vi "CD Init_Prepare Async Data_RT Command Channels.vi"(8 "error in (no error)":errorcluster, 10 "Card Parameters (in)":T1, 11 "Channels In":T6[](array[typedef]) {"RTs"."Mode Codes"."Words Item Refs" format="%.0x"; "RTs"."Mode Codes"."Timestamp Channel Data Reference" format="%.0x"; "RTs"."subAddresses"."Words Item Refs" format="%.0x"; "RTs"."subAddresses"."Timestamp Channel Data Reference" format="%.0x"; "RTs"."Status Channel Data Reference" format="%.0x"; "RTs"."Command Channels Refs" format="%.0x"; "BC"."Acyclic Frames Trigger Channels Refs" format="%.0x"; "BC"."Command Channels Refs" format="%.0x"; "BC"."messages"."Timestamp Channel Data Reference" format="%.0x"; "BC"."messages"."Status Channel Data Refs" format="%.0x"; "BC"."messages"."Words Item Refs" format="%.0x"; "BC"."messages"."Words Block Data Refs"."Data Reference" format="%.0x"}) -> (0 "error out":errorcluster, 3 "Map (RT Command Channels)":T3[](array[typedef]) {"RT Command Channel Ref" format="%.0x"})   [LabVIEW 2017, in "Ballard MIL-1553 Engine.lvlib"]
doc: "This VI creates a static association between NI-VS FIFO Channel Index and Physical Channel, Label Index, Parameter Index for Parameter Channel of a Tx Scheduled Label."
uses:
  Ballard MIL-1553 Engine.lvlib
  Shared/Controls and Global/RT Channel.ctl
  Shared/Controls and Global/RT BC.ctl
  <vilib>/NI Veristand/Custom Device API/Custom Device Item Ref.ctl
  Shared/Controls and Global/RT Message.ctl
  Shared/Controls and Global/RT messageType.ctl
  Shared/Controls and Global/RT CWD1.ctl
  Shared/Controls and Global/RT CWD2.ctl
  <vilib>/NI Veristand/Custom Device API/Data Reference.ctl
  <vilib>/NI Veristand/Custom Device API/Block Data Reference.ctl
  Shared/Controls and Global/RT Remote Terminal.ctl
  Shared/Controls and Global/RT Remote Terminal_rtMode.ctl
  Shared/Controls and Global/RT Remote Terminal_RT subAddress.ctl
  Shared/Controls and Global/RT Remote Terminal_RT direction.ctl
  Shared/Controls and Global/RT Remote Terminal_RT Mode Code.ctl
  Controls/RT Async_Map RT Command Channels.ctl
  Controls/RT Async_Map_Type.ctl
  Controls/Card Parameters.ctl
  Shared/Controls and Global/Initialization Method.ctl
  <vilib>/NI VeriStand/Custom Device API/Custom Device API.lvlib
  <instrlib>/BTI1553Lib/BTI1553LV.lvlib
  Shared/Ballard 1553 Shared.lvlib
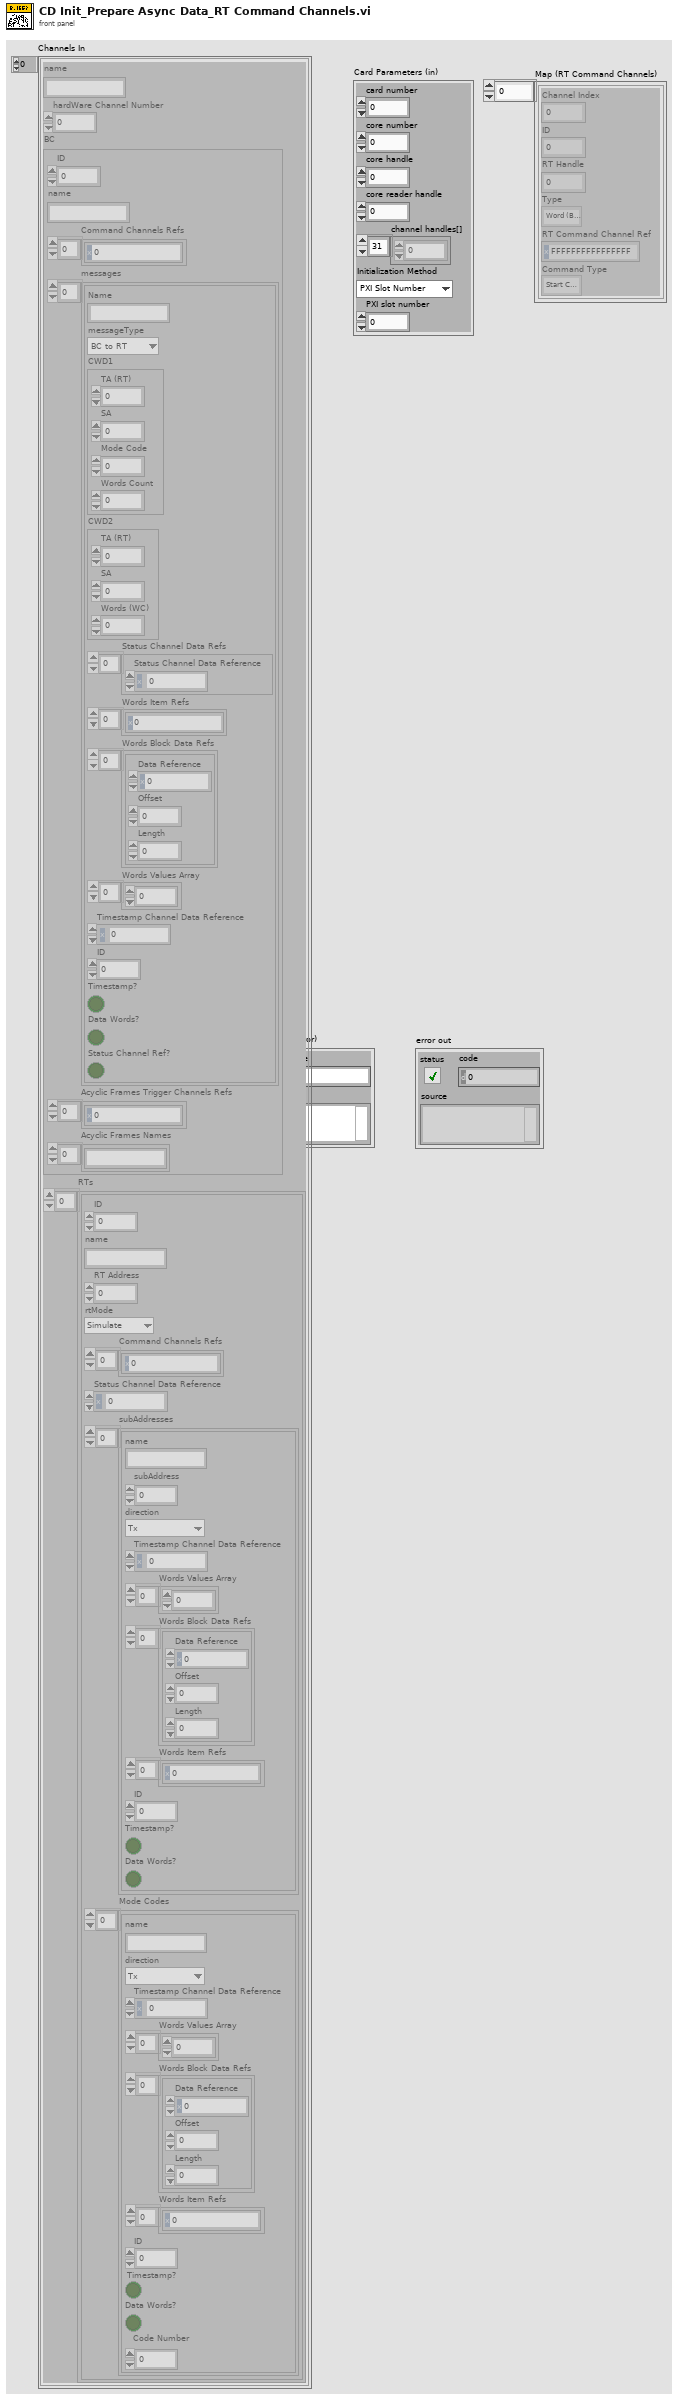
[diagram p1: front panel]
types:
  T1 = typedef "Ballard MIL-1553 Engine.lvlib/Card Parameters.ctl" = cluster{"card number":i32, "core number":i32, "core handle":u64, "core reader handle":u64, "channel handles[]":u64[], "Initialization Method":T2, "PXI slot number":i32}
  T2 = typedef "Ballard 1553 Shared.lvlib/Initialization Method.ctl" = enum16{"PXI Slot Number", "Card Number"}
  T3 = typedef "Ballard MIL-1553 Engine.lvlib/RT Async_Map RT Command Channels.ctl" = cluster{"Channel Index":i32, "ID":i32, "RT Handle":u64, "Type":T4, "RT Command Channel Ref":T5, "Command Type":enum16{"Start Command", "Stop Command"}}
  T4 = typedef "Ballard MIL-1553 Engine.lvlib/RT Async_Map_Type.ctl" = enum16{"Word (BC to RT)", "Word (MC (Rx))", "Acyclic Message Trigger", "Word (RT to ..)", "Word (RT to RT)", "Word (MC (Tx))", "RT Status", "BC Commands", "RT Commands"}
  T5 = typedef "Custom Device API.lvlib/Custom Device Item Ref.ctl" = u64
  T6 = typedef "Ballard 1553 Shared.lvlib/RT Channel.ctl" = cluster{"name":string, "hardWare Channel Number":u16, "BC":T7, "RTs":T14[]}
  T7 = typedef "Ballard 1553 Shared.lvlib/RT BC.ctl" = cluster{"ID":i32, "name":string, "Command Channels Refs":T5[], "messages":T8[], "Acyclic Frames Trigger Channels Refs":T5[], "Acyclic Frames Names":string[]}
  T8 = typedef "Ballard 1553 Shared.lvlib/RT Message.ctl" = cluster{"Name":string, "messageType":T9, "CWD1":T10, "CWD2":T11, "Status Channel Data Refs":T12[], "Words Item Refs":T5[], "Words Block Data Refs":T13[], "Words Values Array":u16[], "Timestamp Channel Data Reference":T12, "ID":i32, "Timestamp?":bool, "Data Words?":bool, "Status Channel Ref?":bool}
  T9 = typedef "Ballard 1553 Shared.lvlib/RT messageType.ctl" = enum16{"BC to RT", "RT to BC", "RT to RT", "MC (Rx)", "MC (Tx)"}
  T10 = typedef "Ballard 1553 Shared.lvlib/RT CWD1.ctl" = cluster{"TA (RT)":i8, "SA":i8, "Mode Code":i8, "Words Count":i8}
  T11 = typedef "Ballard 1553 Shared.lvlib/RT CWD2.ctl" = cluster{"TA (RT)":i8, "SA":i8, "Words (WC)":i8}
  T12 = typedef "Custom Device API.lvlib/Data Reference.ctl" = i32
  T13 = typedef "Custom Device API.lvlib/Block Data Reference.ctl" = cluster{"Data Reference":T12, "Offset":u64, "Length":u64}
  T14 = typedef "Ballard 1553 Shared.lvlib/RT Remote Terminal.ctl" = cluster{"ID":i32, "name":string, "RT Address":i32, "rtMode":T15, "Command Channels Refs":T5[], "Status Channel Data Reference":T12, "subAddresses":T16[], "Mode Codes":T18[]}
  T15 = typedef "Ballard 1553 Shared.lvlib/RT Remote Terminal_rtMode.ctl" = enum16{"Simulate", "Monitor", "Disable"}
  T16 = typedef "Ballard 1553 Shared.lvlib/RT Remote Terminal_RT subAddress.ctl" = cluster{"name":string, "subAddress":i8, "direction":T17, "Timestamp Channel Data Reference":T12, "Words Values Array":u16[], "Words Block Data Refs":T13[], "Words Item Refs":T5[], "ID":i32, "Timestamp?":bool, "Data Words?":bool}
  T17 = typedef "Ballard 1553 Shared.lvlib/RT Remote Terminal_RT direction.ctl" = enum16{"Tx", "Rx"}
  T18 = typedef "Ballard 1553 Shared.lvlib/RT Remote Terminal_RT Mode Code.ctl" = cluster{"name":string, "direction":T17, "Timestamp Channel Data Reference":T12, "Words Values Array":u16[], "Words Block Data Refs":T13[], "Words Item Refs":T5[], "ID":i32, "Timestamp?":bool, "Data Words?":bool, "Code Number":i32}
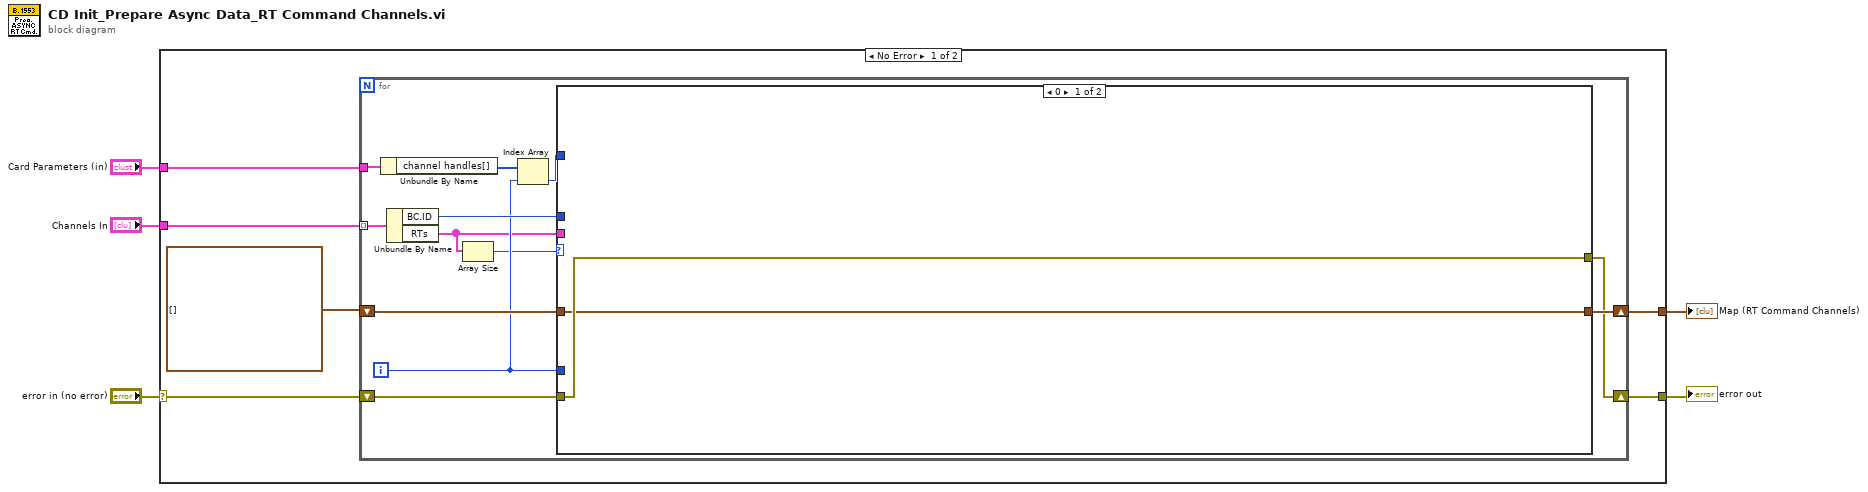
[diagram p0: block diagram]
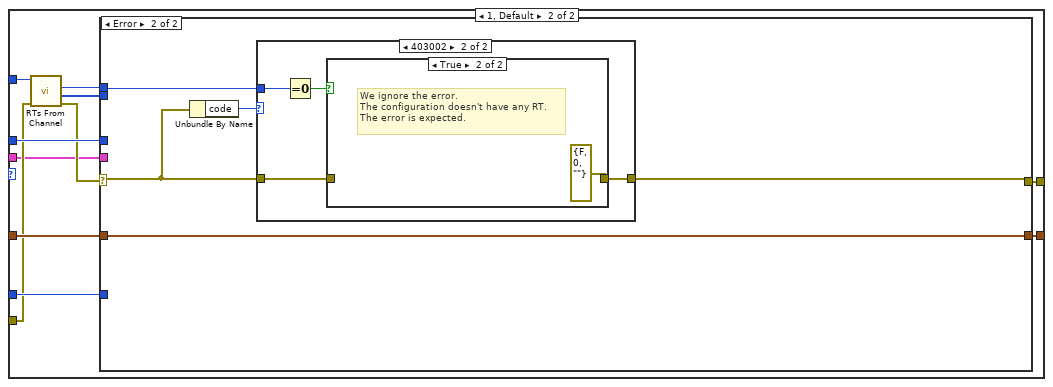
[diagram p2: hidden frame]
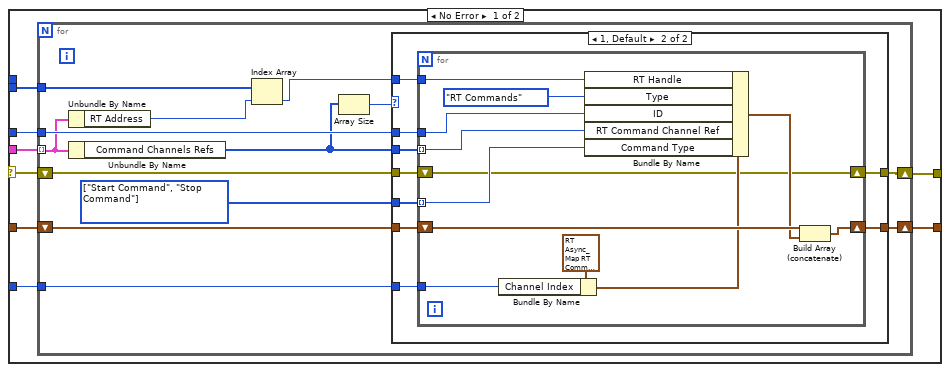
[diagram p3: hidden frame]
diagram:
  n1 = case shown="No Error" "error in (no error)" {
    selector: "error in (no error)" -> [w7 w93]
    tunnel: [w6 w93] -> w4
    tunnel: "Channels In" -> [w11 _]
    tunnel: [w9 _] -> w2
    tunnel: "Card Parameters (in)" -> [w8 _]
    frame No Error {
      n2 = for {
        tunnel: w11 -> [w22] mode=indexing
        shift-right: [w20] -> w9
        shift-left: T3[] [] -> [w21]
        tunnel: w8 -> [w19]
        shift-right: [w16] -> w6
        shift-left: w7 -> [w14]
        i -> [w17]
        n3 = Unbundle By Name(w19) -> ("channel handles[]"=w18:u64[])
        n4 = Unbundle By Name(w22) -> ("BC.ID"=w23:i32, "RTs"=w13:T14[])
        n5 = Array Size(array=w13) -> (size(s)=w12:i32)
        n6 = Index Array(array=w18, index=w17) -> (element=w15:u64)
        n7 = case shown="0" w12 {
          tunnel: w23 -> [_ w36]
          tunnel: w21 -> [w24 w35]
          tunnel: [w24 w34] -> w20
          tunnel: w17 -> [_ w33]
          tunnel: [w25 w32] -> w16
          tunnel: w15 -> [_ w31]
          tunnel: w14 -> [w25 w30]
          tunnel: w13 -> [_ w26]
          frame 0 {
          }
          frame 1, Default {
            n8 = call <instrlib>:"RTs From Channel.vi"("error in (no error)"=w30, "channel handle in"=w31) -> ("error out"=w28:errorcluster, "remote terminal handles out"=w29:u64[], "remote terminal count out"=w27:i32)  [unwired: 6 in, 1 out]
            n9 = case shown="Error" w28 {
              selector: w28 -> [w37 w82]
              tunnel: w36 -> [w44 _]
              tunnel: w35 -> [w43 w85]
              tunnel: [w42 w85] -> w34
              tunnel: w33 -> [w41 _]
              tunnel: [w40 w81] -> w32
              tunnel: w26 -> [w39 _]
              tunnel: w29 -> [w38 _]
              tunnel: w27 -> [_ w83]
              frame No Error {
                n10 = for {
                  tunnel: w44 -> [w54]
                  shift-right: [w56] -> w42
                  shift-left: w43 -> [w55]
                  tunnel: w41 -> [w57]
                  shift-right: [w52] -> w40
                  shift-left: w37 -> [w53]
                  tunnel: w39 -> [w46] mode=indexing
                  tunnel: w38 -> [w48]
                  w49 = enum16{"Start Command", "Stop Command"}[] [enum."Start Command", enum."Stop Command"] items=["Start Command", "Stop Command"]
                  n11 = Unbundle By Name(w46) -> ("RT Address"=w45:i32)
                  n12 = Unbundle By Name(w46) -> ("Command Channels Refs"=w51:T5[])
                  n13 = Index Array(array=w48, index=w45) -> (element=w47:u64)
                  n14 = Array Size(array=w51) -> (size(s)=w50:i32)
                  n15 = case shown="1, Default" w50 {
                    tunnel: w57 -> [_ w68]
                    tunnel: [w59 w67] -> w56
                    tunnel: w55 -> [w59 w66]
                    tunnel: w54 -> [_ w65]
                    tunnel: w47 -> [_ w64]
                    tunnel: w53 -> [w58 w63]
                    tunnel: [w58 w62] -> w52
                    tunnel: w51 -> [_ w61]
                    tunnel: w49 -> [_ w60]
                    frame 0 {
                    }
                    frame 1, Default {
                      n16 = for {
                        tunnel: w68 -> [w80]
                        tunnel: w65 -> [w73]
                        tunnel: w64 -> [w72]
                        tunnel: w61 -> [w71] mode=indexing
                        shift-right: [w69] -> w62
                        shift-left: w63 -> [w69]
                        tunnel: w60 -> [w70] mode=indexing
                        shift-right: [w79] -> w67
                        shift-left: w66 -> [w78]
                        n17 = Bundle By Name(cluster=T3 {"Channel Index"=0, "ID"=0, "RT Handle"=0, "Type"=enum."Word (BC to RT)", "RT Command Channel Ref"=18446744073709551615, "Command Type"=enum."Start Command"} ("Association"), "Channel Index"=w80) -> (w77:T3)
                        n18 = Bundle By Name(cluster=w77, "RT Handle"=w72, "Type"=RT_Async_Map_Type."RT Commands", "ID"=w73, "RT Command Channel Ref"=w71, "Command Type"=w70) -> (w75:T3)
                        n19 = Build Array (concatenate)(w78, w75) -> (w79:T3[])
                      }
                    }
                  }
                }
              }
              frame Error {
                n20 = Unbundle By Name(w82) -> ("code"=w84:i32)
                n21 = case shown="403002" w84 {
                  tunnel: w82 -> [w86 w88]
                  tunnel: w83 -> [_ w90]
                  tunnel: [w86 w87] -> w81
                  frame 0, Default {
                  }
                  frame 403002 {
                    n22 = Equal To 0?(x=w90) -> (x = 0?=w89:bool)
                    n23 = case shown="True" w89 {
                      tunnel: w88 -> [w91 _]
                      tunnel: [w91 errorcluster {"status"=FALSE, "code"=0, "source"=""} ("error IO")] -> w87
                      frame False {
                      }
                      frame True {
                        # "We ignore the error.\nThe configuration doesn't have any RT.\nThe error is expected."
                      }
                    }
                  }
                }
              }
            }
          }
        }
      }
    }
    frame Error {
    }
  }
  "error out" <- w4
  "Map (RT Command Channels)" <- w2
